vi "Vin_Vout_Calc.vi"(0 "aDATA":u8[](array[numeric])) -> (1 "CH R":u8, 2 "V in":dbl, 3 "V Out":dbl)   [LabVIEW 2017]
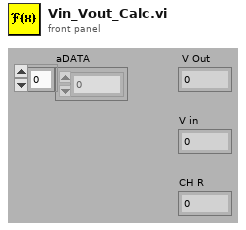
[diagram p1: front panel]
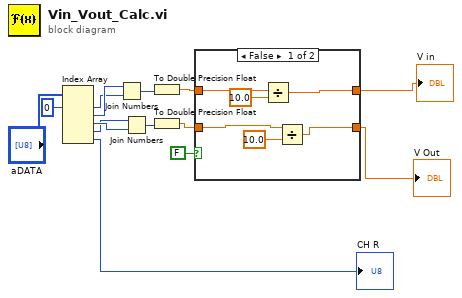
[diagram p0: block diagram]
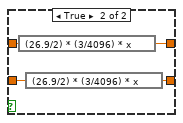
[diagram p2: hidden frame]
diagram:
  n1 = Index Array(array="aDATA", index #1=0 ("index")) -> (element #1=w11:u8, element #2=w12:u8, element #3=w14:u8, element #4=w13:u8, element #5=→"CH R":u8)  [unwired: 4 in]
  n2 = Join Numbers(hi=w12, lo=w11) -> ((hi.lo)=w8:u16)
  n3 = Join Numbers(hi=w13, lo=w14) -> ((hi.lo)=w7:u16)
  n4 = To Double Precision Float(number=w8) -> (double precision float=w5:dbl)
  n5 = To Double Precision Float(number=w7) -> (double precision float=w6:dbl)
  n6 = case shown="False" FALSE {
    tunnel: w6 -> [w16 w24]
    tunnel: w5 -> [w19 w23]
    tunnel: [w15 w22] -> w4
    tunnel: [w20 w21] -> w3
    frame False {
      n7 = Divide(x=w19, y=10.0) -> (x/y=w20:dbl)
      n8 = Divide(x=w16, y=10.0) -> (x/y=w15:dbl)
    }
    frame True {
      n9 = expression code="(26.9/2) * (3/4096) * x"(w23) -> (w21:dbl)
      n10 = expression code="(26.9/2) * (3/4096) * x"(w24) -> (w22:dbl)
    }
  }
  "V in" <- w3
  "V Out" <- w4
